vi "SeCrTs-AI_V_Read_.vi"(7 "Data FIFO Ref":T1, 8 "error in":errorcluster, 10 "number of samples per channel":i32=51, 11 "AI_V_Task":refnum<k21>) -> (0 "error out":errorcluster, 3 "AI_V_Task":refnum<k21>)   [LabVIEW 2022 SP3]
uses:
  RT Controls/SeCrTs-Data FIFO.ctl
  <vilib>/Platform/TimedLoop/XDataNode/timing_clust.ctl
  <vilib>/Platform/TimedLoop/XDataNode/nitl_modes.ctl
  <vilib>/Platform/TimedLoop/XDataNode/wakeup.ctl
  RT Controls/SeCrTs-FGV Read write.ctl
  <vilib>/DAQmx/read.llb/DAQmx Read (Analog 1D Wfm NChan NSamp).vi
  <vilib>/DAQmx/miscellaneous.llb/DAQmx Fill In Error Info.vi
  <vilib>/platform/TimedLoop/XDataNode/XDataNode.xnode
  <vilib>/Platform/TimedLoop/XDataNode/XDNodeRunTimeDep.lvlib
panel:
  out "overflow? 2":bool
  out "overflow?":bool
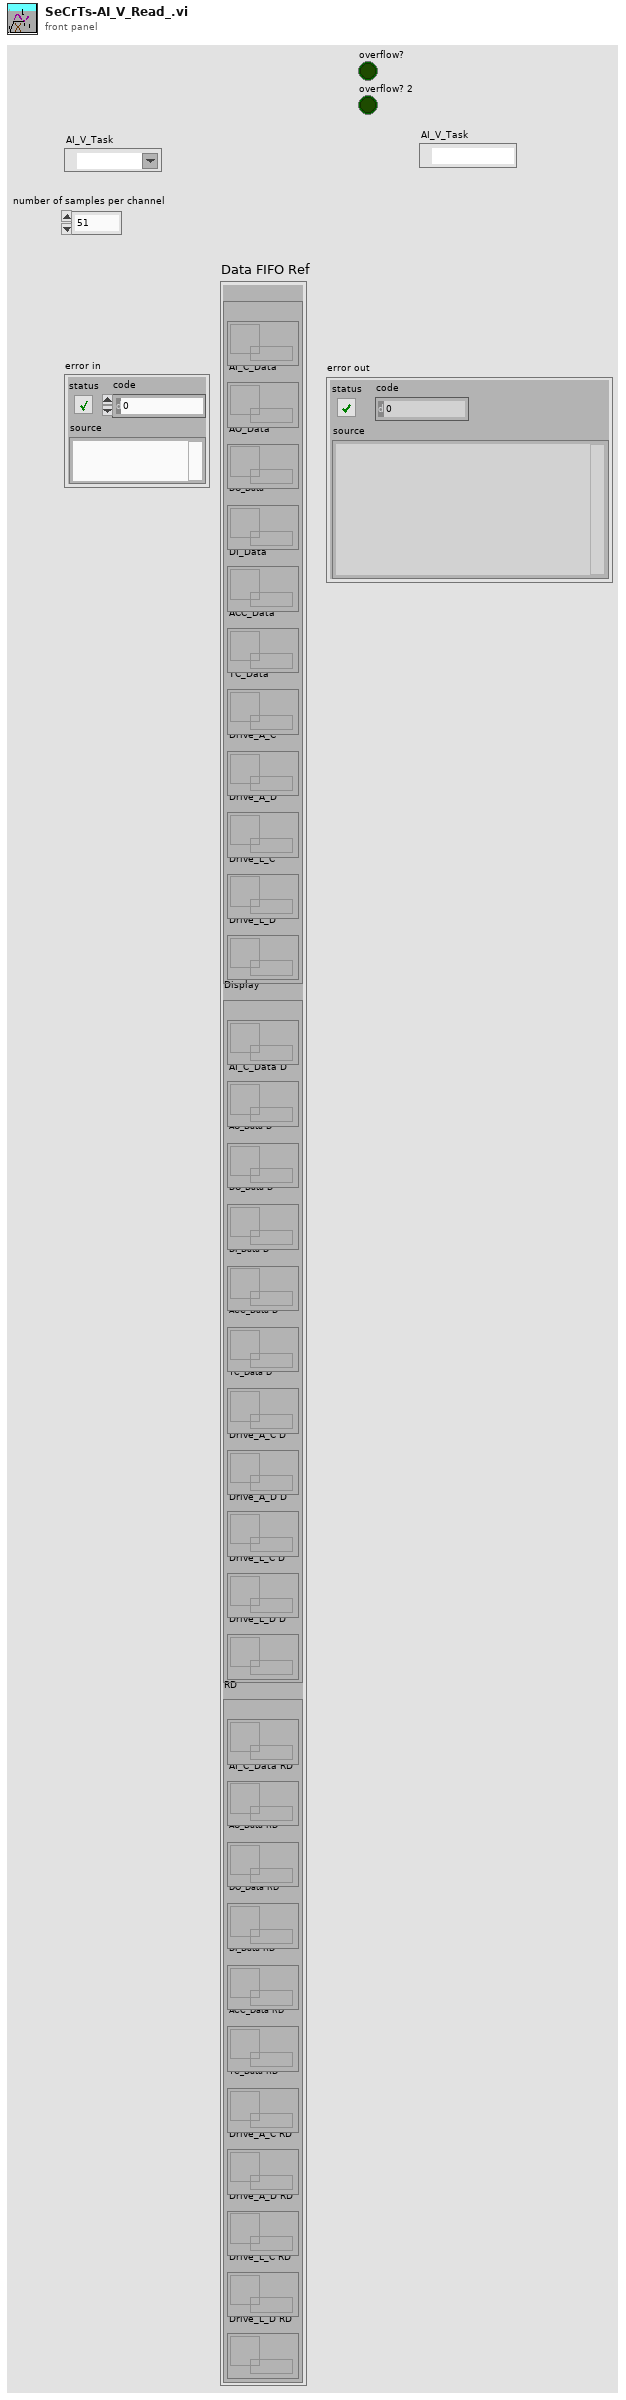
[diagram p1: front panel]
types:
  T1 = typedef "SeCrTs-Data FIFO.ctl" = cluster{"Control":cluster{"AI_V_Data":refnum<queue>, "AI_C_Data":refnum<queue>, "AO_Data":refnum<queue>, "DO_Data":refnum<queue>, "DI_Data":refnum<queue>, "ACC_Data":refnum<queue>, "TC_Data":refnum<queue>, "Drive_A_C":refnum<queue>, "Drive_A_D":refnum<queue>, "Drive_L_C":refnum<queue>, "Drive_L_D":refnum<queue>}, "Display":cluster{"AI_V_Data D":refnum<queue>, "AI_C_Data D":refnum<queue>, "AO_Data D":refnum<queue>, "DO_Data D":refnum<queue>, "DI_Data D":refnum<queue>, "ACC_Data D":refnum<queue>, "TC_Data D":refnum<queue>, "Drive_A_C D":refnum<queue>, "Drive_A_D D":refnum<queue>, "Drive_L_C D":refnum<queue>, "Drive_L_D D":refnum<queue>}, "RD":cluster{"AI_V_Data RD":refnum<queue>, "AI_C_Data RD":refnum<queue>, "AO_Data RD":refnum<queue>, "DO_Data RD":refnum<queue>, "DI_Data RD":refnum<queue>, "ACC_Data RD":refnum<queue>, "TC_Data RD":refnum<queue>, "Drive_A_C RD":refnum<queue>, "Drive_A_D RD":refnum<queue>, "Drive_L_C RD":refnum<queue>, "Drive_L_D RD":refnum<queue>}}
  T2 = cluster{"AO config":cluster{"Channel_Name":string, "Channel_Number":string, "Default_Value":dbl, "Units":string}[], "AI config":cluster{"Channel_Name":string, "Channel_Number":string, "Pre_Scale_min":dbl, "Pre_Scale_max":dbl, "Sensor_min":dbl, "Sensor_max":dbl, "Units":string}[], "DI config":cluster{"Channel_Name":string, "Channel_Number":string, "Default_Value":bool, "DI invert?":bool}[], "DO config":cluster{"Channel_Name":string, "Channel_Number":string, "Default_Value":bool, "DO invert?":bool}[], "TC config":cluster{"Channel_Name":string, "Channel_Number":string, "Pre_Scale_min":dbl, "Pre_Scale_max":dbl, "units":i32, "thermocouple type":i32}[], "ACC config":cluster{"Channel_Name":string, "Channel_Number":string, "Pre_Scale_min":dbl, "Pre_Scale_max":dbl, "Terminal configuration":i32, "Sensitivity":dbl, "Sensitivity units":i32}[], "SG config":cluster{"Channel_Name":string, "Channel_Number":string, "Pre_Scale_min":dbl, "Pre_Scale_max":dbl}[], "Strain Gauge Settings":cluster{"poisson ratio":dbl, "nominal gage resistance":dbl, "gage factor":dbl}, "Bridge Settings":cluster{"voltage excitation value":dbl, "voltage excitation source":i32, "initial bridge voltage":dbl, "lead wire resistance":dbl, "strain configuration":i32}, "Sample Rate":cluster{"AI Sample Rate":dbl[], "AO Sample Rate":dbl[], "DI Sample Rate":dbl[], "TC Sample Rate":dbl[], "DO Sample Rate":dbl[], "SG Sample Rate":dbl[], "ACC Sample Rate":dbl[]}}
  T3 = cluster{"Channel_Name":string, "Channel_Number":string, "Pre_Scale_min":dbl, "Pre_Scale_max":dbl, "Sensor_min":dbl, "Sensor_max":dbl, "Units":string}[]
  T4 = typedef "XDNodeRunTimeDep.lvlib/timing_clust.ctl" = cluster{"Expected End [f-1]":u64, "Actual End [f-1]":u64, "Finished Late? [f-1]":bool, "Expected End [i-1]":u64, "Actual End [i-1]":u64, "Finished Late? [i-1]":bool, "Expected Start [i]":u64, "Actual Start [i]":u64, "Expected Start [f]":u64, "Actual Start [f]":u64, "Source Name":string, "Structure Name":string, "Period":i64, "Deadline":i64, "Offset":i64, "Start":i64, "Priority":i32, "Timeout":i32, "Mode":T5, "Wakeup Reason":T6, "Error":errorcluster, "Source Type":string, "Secondary Source Type":string, "Global End Time":u64, "Global Start Time":u64, "Frame Duration":u64, "Iteration Duration":u64, "Assigned CPU":i32, "I/O Scan Engine Mode":u32}
  T5 = typedef "XDNodeRunTimeDep.lvlib/nitl_modes.ctl" = enum32{"No Change", "Process missed periods, maintain original phase", "Discard missed periods, maintain original phase", "Process missed periods, ignore original phase", "Discard missed periods, ignore original phase"}
  T6 = typedef "XDNodeRunTimeDep.lvlib/wakeup.ctl" = enum32{"Normal", "Aborted", "Asynchronous wakeup", "Timing source error", "Timed loop error", "Timeout"}
  T7 = typedef "SeCrTs-FGV Read write.ctl" = enum16{"Write", "Read"}
  T8 = enum16{"AI C", "AI V", "AO", "DI", "DO", "TC", "ACC", "DR L", "DR A"}
  T9 = enum16{"Init", "Read 'All'", "Read 'n'", "Read '1'", "Write '1'", "Write 'n'", "Write 'All'"}
  T10 = cluster{"Start DAQ":bool, "Stop DAQ":bool, "RT Stop":bool, "RT Exit":bool, "Start Seq":bool}
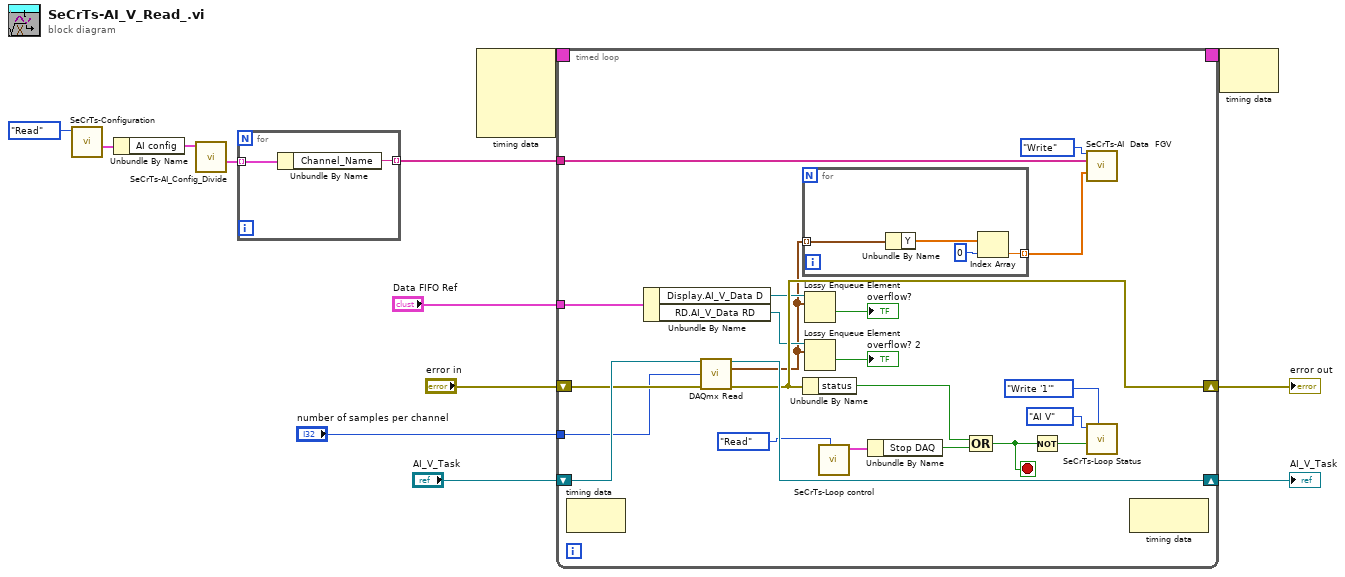
[diagram p0: block diagram]
diagram:
  n1 = call "SeCrTs-Configuration.vi"("Enum"=enum16{"Write", "Read"}."Read") -> ("Config out"=w4:T2)  [unwired: 10 in]
  n2 = Unbundle By Name(w4) -> ("AI config"=w3:T3)
  n3 = call "SeCrTs-AI_Config_Divide.vi"("AI config"=w3) -> ("AI C"=w2:T3)  [unwired: 9 in, 1 out]
  n4 = for {
    tunnel: w2 -> [w15] mode=indexing
    tunnel: [w14] -> w1 mode=indexing
    n5 = Unbundle By Name(w15) -> ("Channel_Name"=w14:string)
  }
  n6 = node-c288() -> (w8:T4)  [unwired: 4 in]
  n7 = timed-loop {
    shift-right: [w35] -> w6
    shift-left: "AI_V_Task" -> [w37]
    shift-right: [w34] -> w11
    shift-left: "error in" -> [w36]
    tunnel: "number of samples per channel" -> [w32]
    tunnel: "Data FIFO Ref" -> [w27]
    timing: w8 -> [_]
    timing-out: [_] -> w7
    tunnel: w1 -> [w18]
    stop <- w33 stop-if-true
    n8 = node-c288() -> ()  [unwired: 1 in, 1 out]
    n9 = Unbundle By Name(w27) -> ("Display.AI_V_Data D"=w23:refnum<queue>, "RD.AI_V_Data RD"=w22:refnum<queue>)
    n10 = call-poly <vilib>:"DAQmx Read.vi"("task/channels in"=w37, "number of samples per channel"=w32, "error in"=w36) -> ("task out"=w35:refnum<k21>, "data"=w20:waveform(dbl)[], "error out"=w34:errorcluster)  [unwired: 10 in]
    n11 = for {
      tunnel: [w40] -> w21 mode=indexing
      tunnel: w20 -> [w38] mode=indexing
      n12 = Unbundle By Name(w38) -> ("Y"=w41:dbl[])
      n13 = Index Array(array=w41, index=0) -> (element=w40:dbl)
    }
    n14 = Unbundle By Name(w34) -> ("status"=w31:bool)
    n15 = Lossy Enqueue Element(queue=w23, element=w20) -> (overflow?=→"overflow?":bool)  [unwired: 1 in, 3 out]
    n16 = Lossy Enqueue Element(queue=w22, element=w20) -> (overflow?=→"overflow? 2":bool)  [unwired: 1 in, 3 out]
    n17 = call "SeCrTs-Loop control.vi"("Action"=enum16{"Init", "Write", "Read"}."Read") -> ("Loop Control out"=w30:T10)  [unwired: 9 in, 1 out]
    n18 = Unbundle By Name(w30) -> ("Stop DAQ"=w29:bool)
    n19 = Compound Arithmetic op=OR(w31, w29) -> (w33:bool)
    n20 = Not(x=w33) -> (.not. x?=w24:bool)
    n21 = call "SeCrTs-AI  Data  FGV.vi"("Write/Read"=SeCrTs-FGV_Read_write."Write", "AI Channels Name LP"=w18, "AI Y LP data"=w21) -> ()  [unwired: 9 in, 4 out]
    n22 = call "SeCrTs-Loop Status.vi"("Option"=T9."Write '1'", "Status"=w24, "Loop"=T8."AI V") -> ()  [unwired: 6 in, 3 out]
    n23 = node-c288() -> ()  [unwired: 1 in, 1 out]
  }
  "error out" <- w11
  "AI_V_Task" <- w6
  n24 = node-c288(w7) -> ()  [unwired: 1 out]
